vi "NumIntegrate_Rk4_Dbl_X.vi"(5 "Func":refnum<vi>, 7 "ExtraData":variant, 8 "DT":dbl, 11 "X":dbl) -> (0 "Error":bool, 3 "Integral":dbl)   [LabVIEW 2019, in "Trajectory_Library.lvlib"]
doc: "NOT DONE"
uses:
  Trajectory_Library.lvlib
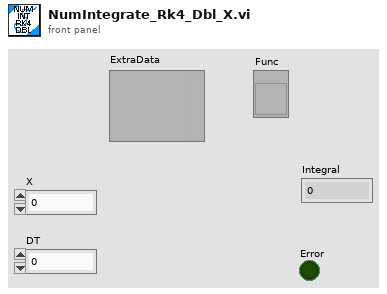
[diagram p1: front panel]
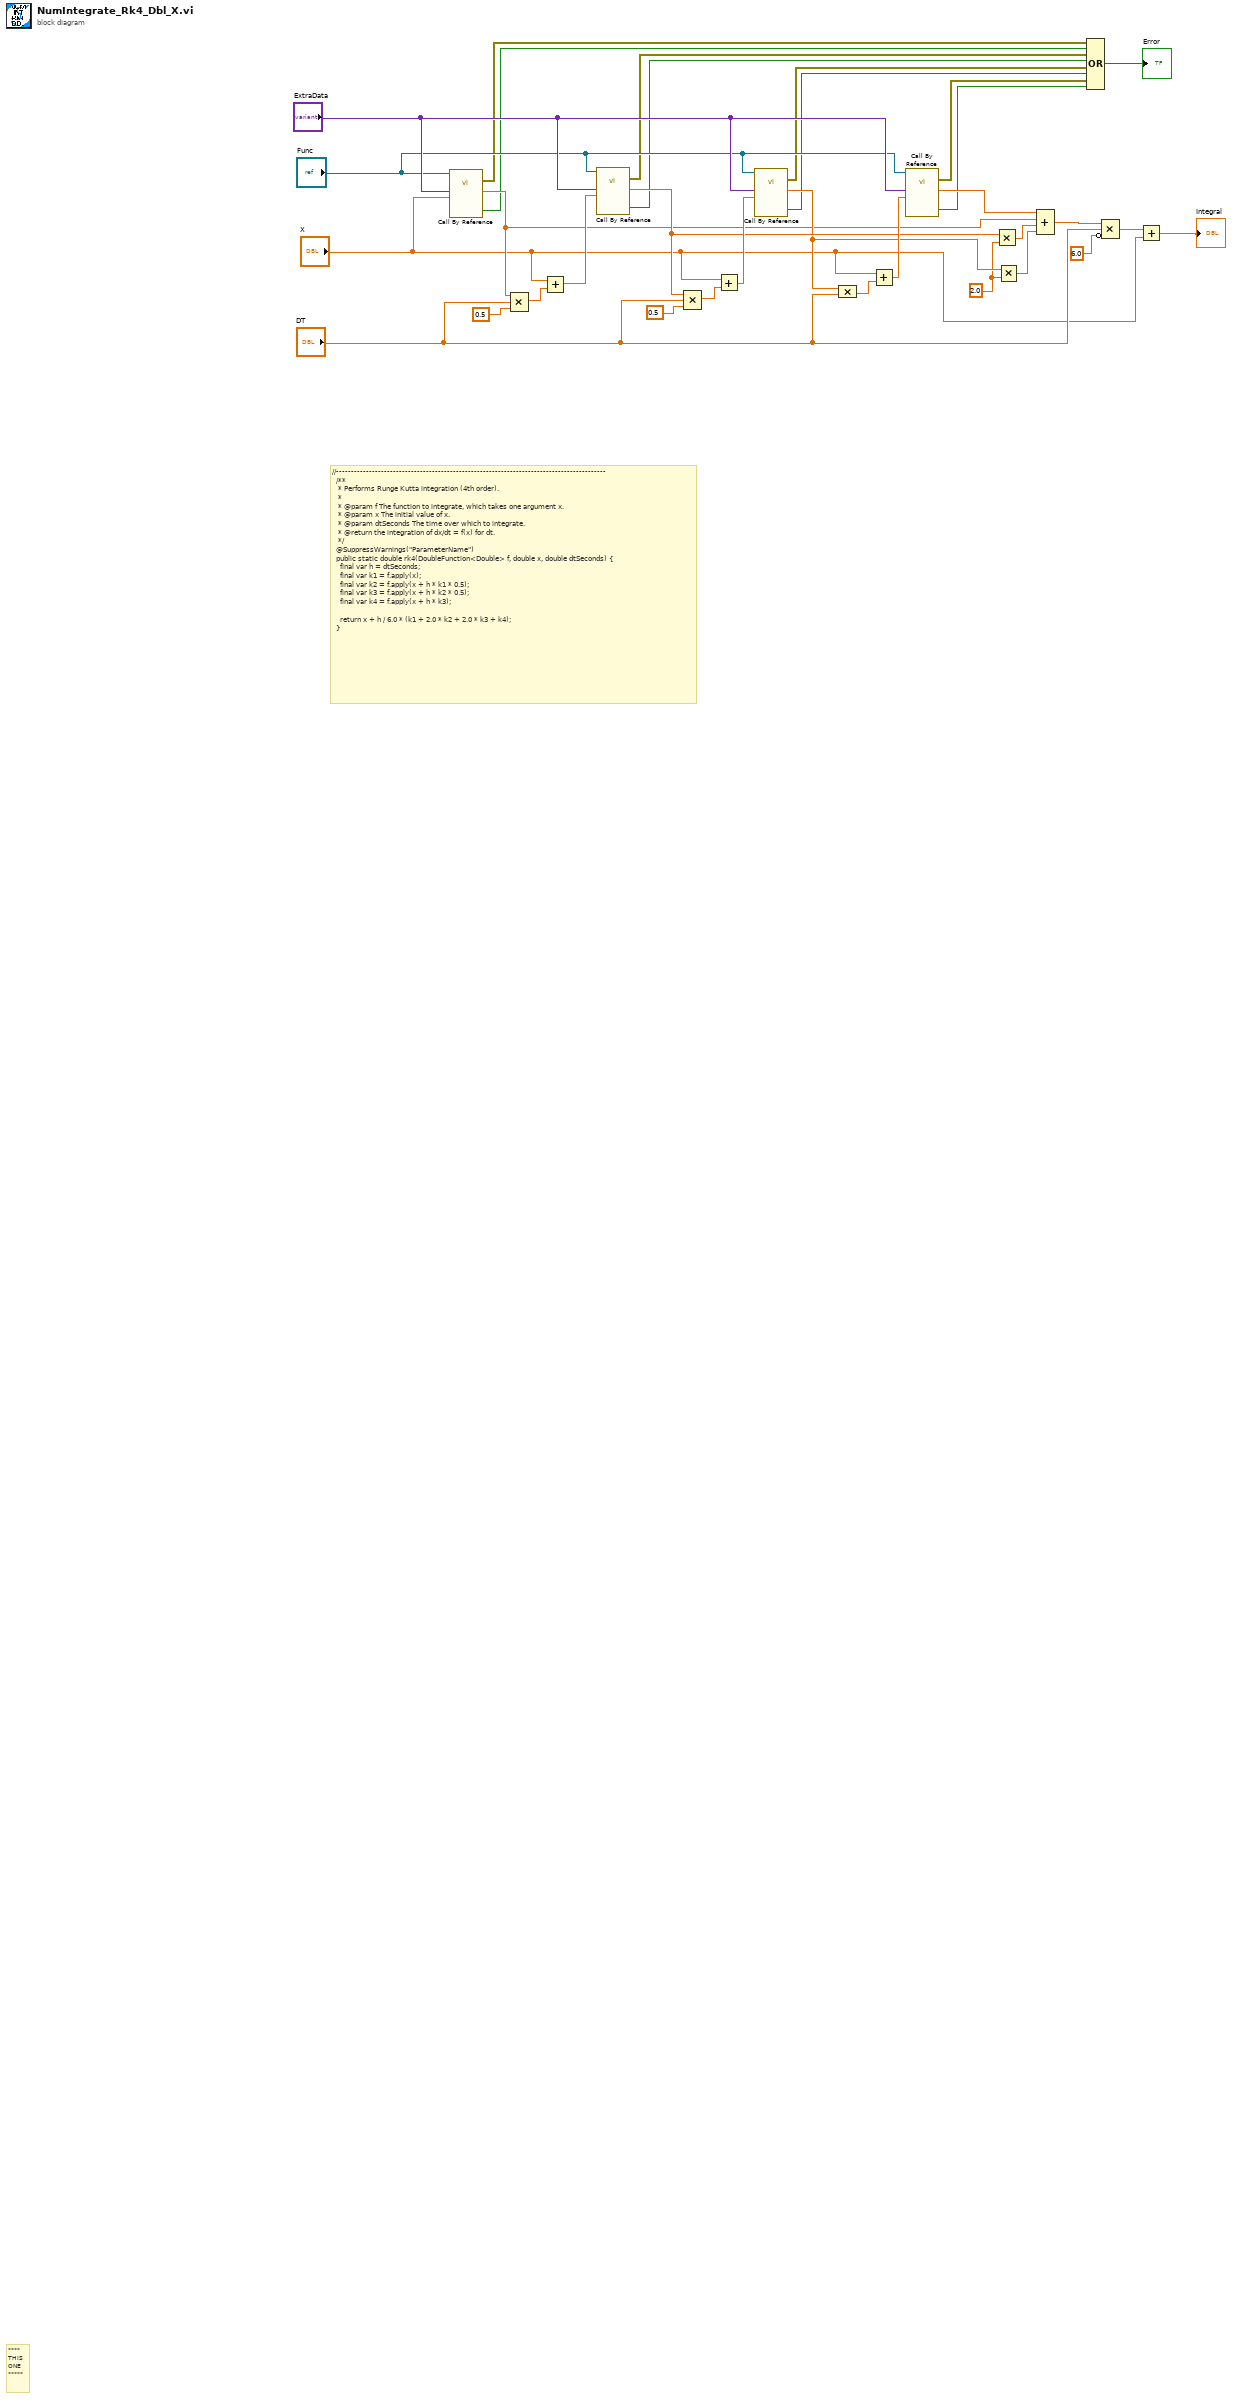
[diagram p0: block diagram]
diagram:
  w19 = 2.0 ("y")
  # "//------------------------------------------------------------------------------------------\n  /**\n   * Performs Runge Kutta integration (4th order).\n   *\n   * @param f The function to integrate, which takes one argument x.\n   * @param x The initial value of x.\n   * @param dtSeconds The time over which to integrate.\n   * @return the integration of dx/dt = f(x) for dt.\n   */\n  @SuppressWarnings(\"ParameterName\")\n  public static double rk4(DoubleFunction<Double> f, double x, double dtSeconds) {\n    final var h = dtSeconds;\n    final var k1 = f.apply(x);\n    final var k2 = f.apply(x + h * k1 * 0.5);\n    final var k3 = f.apply(x + h * k2 * 0.5);\n    final var k4 = f.apply(x + h * k3);\n\n    return x + h / 6.0 * (k1 + 2.0 * k2 + 2.0 * k3 + k4);\n  }"
  # "****\nTHIS\nONE\n*****"
  n1 = call-by-ref "?"(reference="Func", "X"="X", "Variant"="ExtraData") -> (error out=w9:errorcluster, "Error"=w8:bool, "NewX"=w21:dbl)  [unwired: 9 in, 1 out]
  n2 = Compound Arithmetic op=MULTIPLY(w21, "DT", 0.5 ("value")) -> (w31:dbl)
  n3 = Add(x="X", y=w31) -> (x+y=w30:dbl)
  n4 = call-by-ref "?"(reference="Func", "X"=w30, "Variant"="ExtraData") -> (error out=w6:errorcluster, "Error"=w5:bool, "NewX"=w23:dbl)  [unwired: 9 in, 1 out]
  n5 = Compound Arithmetic op=MULTIPLY(w23, "DT", 0.5 ("value")) -> (w28:dbl)
  n6 = Add(x="X", y=w28) -> (x+y=w27:dbl)
  n7 = call-by-ref "?"(reference="Func", "X"=w27, "Variant"="ExtraData") -> (error out=w4:errorcluster, "Error"=w3:bool, "NewX"=w22:dbl)  [unwired: 9 in, 1 out]
  n8 = Compound Arithmetic op=MULTIPLY(w22, "DT") -> (w25:dbl)
  n9 = Add(x="X", y=w25) -> (x+y=w24:dbl)
  n10 = call-by-ref "?"(reference="Func", "X"=w24, "Variant"="ExtraData") -> (error out=w2:errorcluster, "Error"=w1:bool, "NewX"=w20:dbl)  [unwired: 9 in, 1 out]
  n11 = Multiply(x=w23, y=w19) -> (x*y=w18:dbl)
  n12 = Multiply(x=w22, y=w19) -> (x*y=w17:dbl)
  n13 = Compound Arithmetic op=ADD(w20, w21, w18, w17) -> (w16:dbl)
  n14 = Compound Arithmetic op=OR(w9, w8, w6, w5, w4, w3, w2, w1) -> (→"Error":bool)
  n15 = Compound Arithmetic op=MULTIPLY(w16, "DT", invert 6.0 ("y")) -> (w13:dbl)
  n16 = Add(x=w13, y="X") -> (x+y=→"Integral":dbl)
